vi "Find Available Tests (SubVI).vi"(0 "References":T1) -> ()   [LabVIEW 2010]
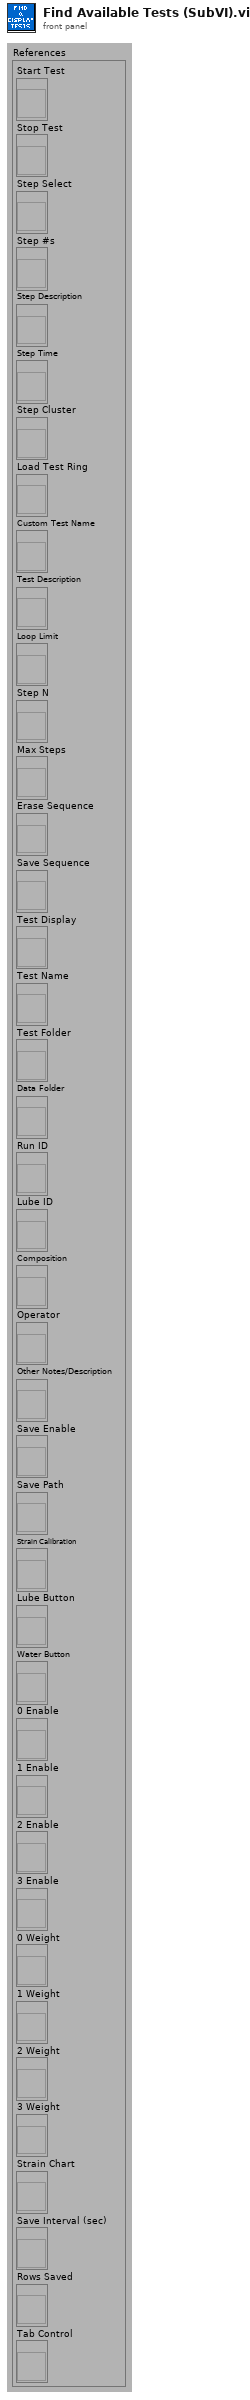
[diagram p1: front panel]
types:
  T1 = cluster{"Start Test":refnum<vi>, "Stop Test":refnum<vi>, "Step Select":refnum<vi>, "Step #s":refnum<vi>, "Step Description":refnum<vi>, "Step Time":refnum<vi>, "Step Cluster":refnum<vi>, "Load Test Ring":refnum<vi>, "Custom Test Name":refnum<vi>, "Test Description":refnum<vi>, "Loop Limit":refnum<vi>, "Step N":refnum<vi>, "Max Steps":refnum<vi>, "Erase Sequence":refnum<vi>, "Save Sequence":refnum<vi>, "Test Display":refnum<vi>, "Test Name":refnum<vi>, "Test Folder":refnum<vi>, "Data Folder":refnum<vi>, "Run ID":refnum<vi>, "Lube ID":refnum<vi>, "Composition":refnum<vi>, "Operator":refnum<vi>, "Other Notes/Description":refnum<vi>, "Save Enable":refnum<vi>, "Save Path":refnum<vi>, "Strain Calibration":refnum<vi>, "Lube Button":refnum<vi>, "Water Button":refnum<vi>, "0 Enable":refnum<vi>, "1 Enable":refnum<vi>, "2 Enable":refnum<vi>, "3 Enable":refnum<vi>, "0 Weight":refnum<vi>, "1 Weight":refnum<vi>, "2 Weight":refnum<vi>, "3 Weight":refnum<vi>, "Strain Chart":refnum<vi>, "Save Interval (sec)":refnum<vi>, "Rows Saved":refnum<vi>, "Tab Control":refnum<vi>}
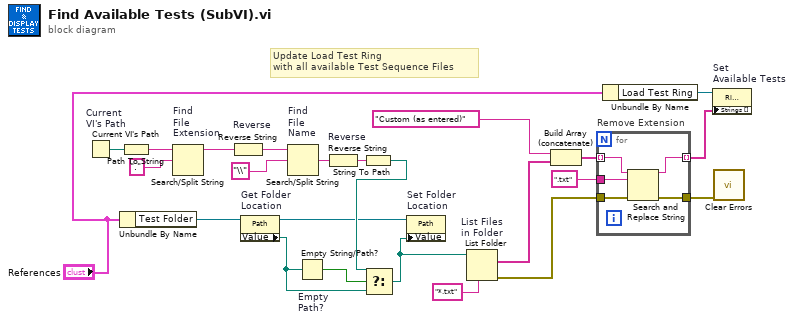
[diagram p0: block diagram]
diagram:
  # "Update Load Test Ring\nwith all available Test Sequence Files"
  n1 = Current VI's Path "Current\nVI's Path"() -> (path=w13:path)
  n2 = Unbundle By Name("References") -> ("Test Folder"=w5:refnum<vi>)
  n3 = Path To String(path=w13) -> (string=w8:string)
  n4 = Search/Split String "Find\nFile \nExtension"(string=w8, search string/char (-)=".") -> (substring before match=w9:string)  [unwired: 1 in, 2 out]
  n5 = Reverse String "Reverse"(1:w9) -> (0:w10:string)
  n6 = property on="Get Folder\nLocation" class="Path"(reference=w5) -> (reference out=w3:refnum<vi>, "Value"=w4:path)  [unwired: 1 in, 1 out]
  n7 = Search/Split String "Find\nFile \nName"(string=w10, search string/char (-)="\\") -> (match + rest of string=w12:string)  [unwired: 1 in, 2 out]
  n8 = Empty String/Path? "Empty\nPath?"(string/path=w4) -> (empty?=w14:bool)
  n9 = Reverse String "Reverse"(1:w12) -> (0:w6:string)
  n10 = String To Path(string=w6) -> (path=w23:path)
  n11 = Select(t=w23, s=w14, f=w4) -> (s? t:f=w2:path)
  n12 = property on="Set Folder\nLocation" class="Path"(reference=w3, "Value"=w2) -> ()  [unwired: 1 in, 2 out]
  n13 = List Folder "List Files\nin Folder"(path=w2, pattern="*.txt") -> (filenames=w22:string[], error out=w18:errorcluster)  [unwired: 1 in, 3 out]
  n14 = Build Array (concatenate)("Custom (as entered)", w22) -> (w20:string[])
  n15 = for "Remove Extension" {
    tunnel: w20 -> [w28] mode=indexing
    tunnel: ".txt" ("pattern") -> [w29]
    tunnel: w18 -> [w27]
    tunnel: [w26] -> w17
    tunnel: [w25] -> w16 mode=indexing
    n16 = Search and Replace String(input string=w28, search string=w29, error in=w27) -> (result string=w25:string, error out=w26:errorcluster)  [unwired: 5 in, 2 out]
  }
  n17 = Unbundle By Name("References") -> ("Load Test Ring"=w1:refnum<vi>)
  n18 = property on="Set\nAvailable Tests" class="Ring (strict)"(reference=w1, "Strings []"=w16) -> ()  [unwired: 1 in, 2 out]
  n19 = call <vilib>:"Clear Errors.vi"("error in (no error)"=w17) -> ()  [unwired: 6 in, 1 out]
